vi "Filter Position.vi"(7 "LabVIEW Web Service Request":refnum<class "Web Request.lvclass">, 11 "Position":bool) -> ()   [LabVIEW 2014]
uses:
  <vilib>/wsapi/Web Request.lvclass
  <vilib>/wsapi/class/subVIs/Write Boolean Session Variable.vi
panel:
  out "previous value":string
  # "Use the Web Service Request input terminal to call the VIs on the Web Services palette. Do not remove it from the connector pane unless you don't need access to the palette."
  # "Each additional control wired to the connector pane will be available as an input in the URL. To include an indicator in terminal-mode output (the default setting), it must also be wired to the connector pane."
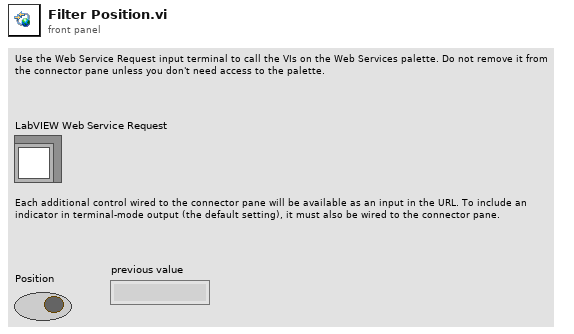
[diagram p1: front panel]
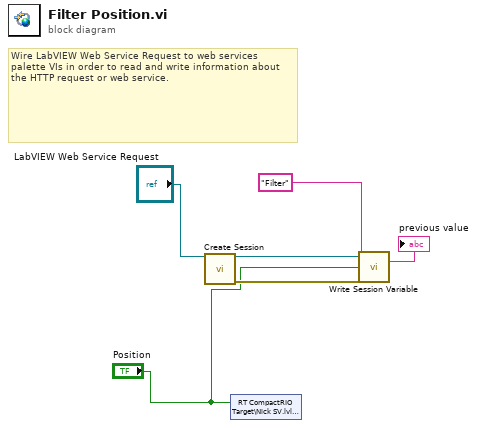
[diagram p0: block diagram]
diagram:
  # "Wire LabVIEW Web Service Request to web services palette VIs in order to read and write information about the HTTP request or web service."
  n1 = call <vilib>:"Create Session.vi"("LabVIEW Web Service Request"="LabVIEW Web Service Request") -> ("LabVIEW Web Service Request out"=w5:refnum<class "Web Request.lvclass">, "error out"=w4:errorcluster)  [unwired: 12 in, 1 out]
  n2 = shared-variable "RT CompactRIO Target\\Nick SV.lvlib\\Filter"("Position") -> ()  [unwired: 1 in, 1 out]
  n3 = call-poly <vilib>:"Write Session Variable.vi"("LabVIEW Web Service Request"=w5, "key"="Filter", "value"="Position", "error in (no error)"=w4) -> ("previous value"=→"previous value":string)  [unwired: 8 in, 3 out]
